vi "Update Previous Step Values.vi"(8 "error in (no error)":errorcluster, 11 "Output Sequencer in":refnum<class "Output Sequencer.lvclass">) -> (0 "error out":errorcluster, 3 "Output Sequencer out":refnum<class "Output Sequencer.lvclass">)   [LabVIEW 2020, in "Output Sequencer.lvlib" / "Output Sequencer.lvclass"]
uses:
  Output Sequencer.lvclass
  Output Sequencer.lvclass/Output Sequencer.ctl
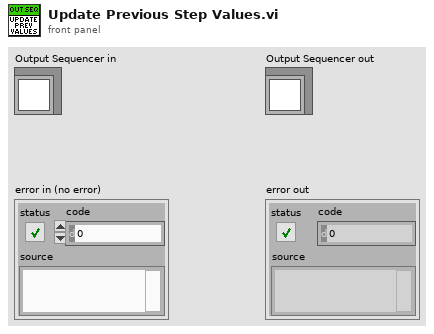
[diagram p1: front panel]
types:
  T1 = typedef "Output Sequencer.lvlib/Output Sequencer.lvclass/Compiled Step.ctl" = cluster{"Precondition":T2, "Duration":dbl, "Mode":string, "Delay Between Values":dbl, "Analog Values":T2[], "Digital Values":T2[], "Postcondition":T2, "On True":string, "On False":string}
  T2 = typedef "Output Sequencer.lvlib/Output Sequencer.lvclass/Expression Data.ctl" = cluster{"Empty?":bool, "Expression":refnum<class "mupExpr.lvclass">, "Variable Names":string[]}
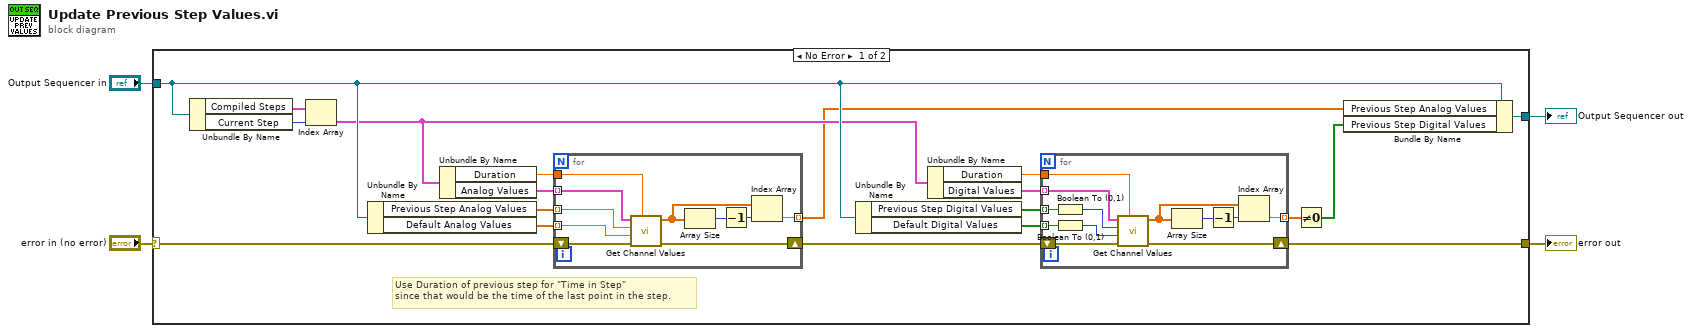
[diagram p0: block diagram]
diagram:
  n1 = case shown="No Error" "error in (no error)" {
    selector: "error in (no error)" -> [w5 w47]
    tunnel: [w23 w46] -> w4
    tunnel: [w22 w47] -> w3
    tunnel: "Output Sequencer in" -> [w21 w46]
    frame No Error {
      # "Use Duration of previous step for \"Time in Step\"\nsince that would be the time of the last point in the step."
      n2 = Unbundle By Name(w21) -> ("Compiled Steps"=w19:T1[], "Current Step"=w18:i32)
      n3 = Index Array(array=w19, index=w18) -> (element=w20:T1)
      n4 = Unbundle By Name(w21) -> ("Previous Step Analog Values"=w15:dbl[], "Default Analog Values"=w14:dbl[])
      n5 = Unbundle By Name(w20) -> ("Duration"=w13:dbl, "Analog Values"=w16:T2[])
      n6 = for {
        tunnel: w16 -> [w30] mode=indexing
        tunnel: [w33] -> w17 mode=indexing
        tunnel: w15 -> [w29] mode=indexing
        tunnel: w14 -> [w27] mode=indexing
        tunnel: w13 -> [w26]
        shift-right: [w24] -> w8
        shift-left: w5 -> [w25]
        n7 = call "Get Channel Values.vi"("Time in Step"=w26, "error in (no error)"=w25, "Default Value"=w27, "Previous Value"=w29, "Channel Value Expression"=w30) -> ("error out"=w24:errorcluster, "Channel Values"=w28:dbl[])  [unwired: 5 in]
        n8 = Array Size(array=w28) -> (size(s)=w32:i32)
        n9 = Decrement(x=w32) -> (x-1=w31:i32)
        n10 = Index Array(array=w28, index=w31) -> (element=w33:dbl)
      }
      n11 = Unbundle By Name(w21) -> ("Previous Step Digital Values"=w7:bool[], "Default Digital Values"=w6:bool[])
      n12 = Unbundle By Name(w20) -> ("Duration"=w12:dbl, "Digital Values"=w11:T2[])
      n13 = for {
        tunnel: w11 -> [w42] mode=indexing
        tunnel: [w45] -> w10 mode=indexing
        tunnel: w12 -> [w40]
        shift-right: [w38] -> w22
        shift-left: w8 -> [w39]
        tunnel: w7 -> [w37] mode=indexing
        tunnel: w6 -> [w34] mode=indexing
        n14 = Boolean To (0,1)(Boolean=w37) -> (0, 1=w36:i16)
        n15 = Boolean To (0,1)(Boolean=w34) -> (0, 1=w35:i16)
        n16 = call "Get Channel Values.vi"("Time in Step"=w40, "error in (no error)"=w39, "Default Value"=w35, "Previous Value"=w36, "Channel Value Expression"=w42) -> ("error out"=w38:errorcluster, "Channel Values"=w41:dbl[])  [unwired: 5 in]
        n17 = Array Size(array=w41) -> (size(s)=w44:i32)
        n18 = Decrement(x=w44) -> (x-1=w43:i32)
        n19 = Index Array(array=w41, index=w43) -> (element=w45:dbl)
      }
      n20 = Not Equal To 0?(x=w10) -> (x != 0?=w9:bool[])
      n21 = Bundle By Name(cluster=w21, "Previous Step Analog Values"=w17, "Previous Step Digital Values"=w9) -> (w23:refnum<class "Output Sequencer.lvclass">)
    }
    frame Error {
    }
  }
  "Output Sequencer out" <- w4
  "error out" <- w3
